vi "3D-十字标Ground.vi"(8 "XY index":cluster{"X":dbl, "Y":dbl}[](array[cluster]), 11 "输入图片":T1(plugin-control)) -> (3 "输出图片":T1(plugin-control))   [LabVIEW 2015]
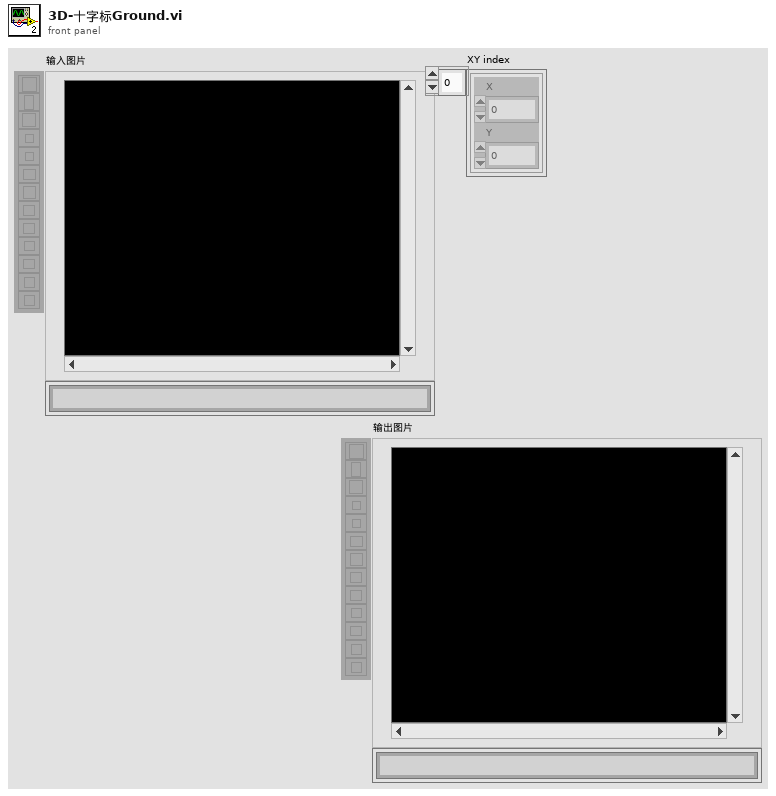
[diagram p1: front panel]
types:
  T1 = typedef "IMAQ Image.ctl" = refnum<image>
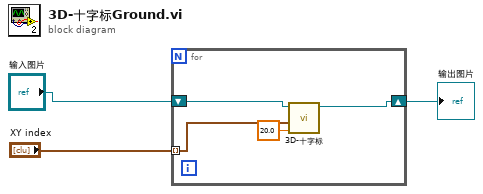
[diagram p0: block diagram]
diagram:
  n1 = for {
    tunnel: "XY index" -> [w5] mode=indexing
    shift-right: [w6] -> w2
    shift-left: "输入图片" -> [w7]
    n2 = call "3D-十字标.vi"("radius"=20.0, "CenterPos"=w5, "输入图片"=w7) -> ("输出图片"=w6:T1)  [unwired: 7 in, 1 out]
  }
  "输出图片" <- w2
